vi "Configure Measurement (Pulse Width).vi"(5 "Pulse Width Reference Level (50 Percent)":dbl=50.0 format="%^#_6g", 8 "error in (no error)":errorcluster, 9 "Pulse Width Type (0:Positive)":i32(ring) items=["Positive", "Negative"], 10 "Channel (1:Channel 1)":i32(ring)=1 items=["Channel 1"=1, "Channel 2"=2], 11 "VISA resource name":refnum<visa-resource-name>) -> (0 "error out":errorcluster, 3 "VISA resource name out":refnum<visa-resource-name>)   [LabVIEW 2024, in "Agilent 532XX Series.lvlib"]
doc: "Configures the settings required for Pulse Width measurements.\n\n<B>Note:</B> This VI only applies to the Agilent 53220A/53230A."
uses:
  Agilent 532XX Series.lvlib
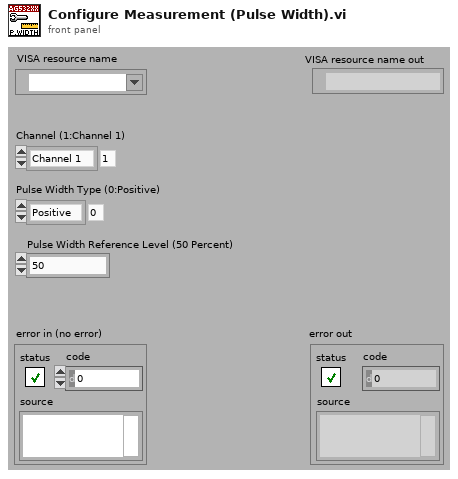
[diagram p1: front panel]
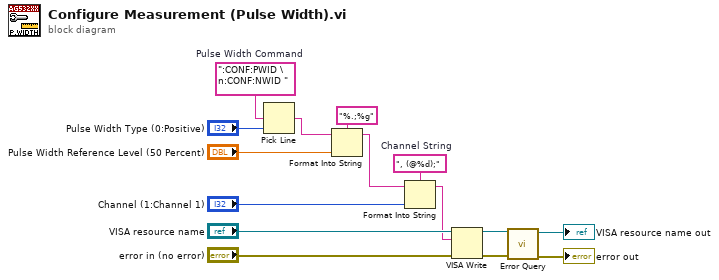
[diagram p0: block diagram]
diagram:
  w3 = ":CONF:PWID \n:CONF:NWID "  # Pulse Width Command
  w11 = ", (@%d);"  # Channel String
  n1 = Pick Line(multi-line string=w3, line index="Pulse Width Type (0:Positive)") -> (output string=w4:string)  [unwired: 1 out]
  n2 = Format Into String(format string="%.;%g", initial string=w4, "Pulse Width Reference Level (50 Percent)") -> (resulting string=w5:string)  [unwired: 1 in, 1 out]
  n3 = Format Into String(format string=w11, initial string=w5, "Channel (1:Channel 1)") -> (resulting string=w6:string)  [unwired: 1 in, 1 out]
  n4 = VISA Write(VISA resource name="VISA resource name", write buffer=w6, error in (no error)="error in (no error)") -> (VISA resource name out=w10:refnum<visa-resource-name>, error out=w8:errorcluster)  [unwired: 1 out]
  n5 = call "Error Query.vi"("error in (no error)"=w8, "VISA resource name"=w10) -> ("error out"=→"error out":errorcluster, "VISA resource name out"=→"VISA resource name out":refnum<visa-resource-name>)  [unwired: 8 out]
